vi "Untitled 402.vi"() -> ()   [LabVIEW 2009]
uses:
  <vilib>/addons/_office/excel.llb/Excel Easy Table (str).vi
  <vilib>/Utility/NIReport.llb/NI_report.lvclass
  <vilib>/addons/_office/NI_ReportGenerationToolkit.lvlib
panel:
  out "next cell top-right":cluster{"row":i32, "column":i32}
  out "next cell bottom-left":cluster{"row":i32, "column":i32}
  in  "error in (no error)":errorcluster
  out "Array":i32[][](array[numeric])
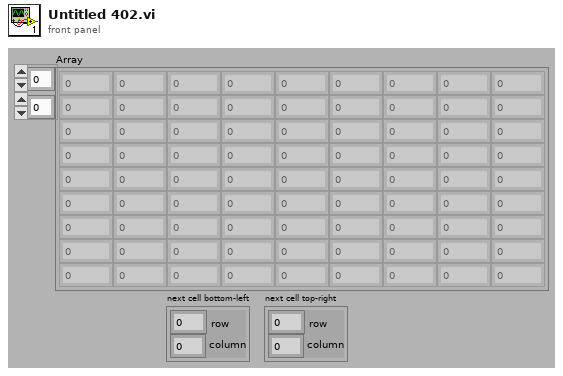
[diagram p1: front panel]
types:
  T1 = enum16{"maximized", "minimized", "normal", "no change"}
  T2 = enum16{"Standard Report", "HTML", "Word", "Excel"}
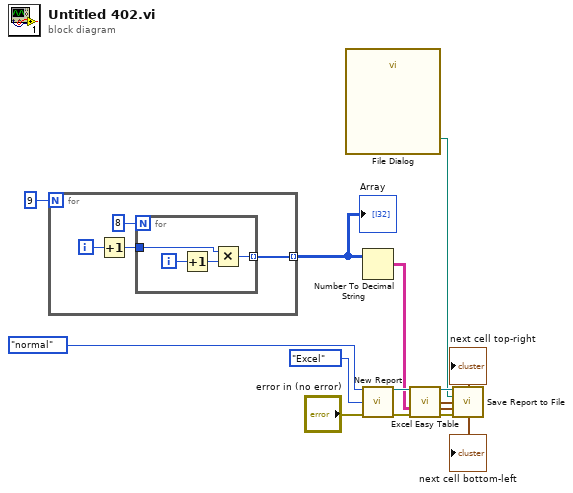
[diagram p0: block diagram]
diagram:
  n1 = for {
    N: 9 -> [_]
    tunnel: [w14] -> w7 mode=indexing
    i -> [w16]
    n2 = Increment(x=w16) -> (x+1=w15:i32)
    n3 = for {
      N: 8 -> [_]
      tunnel: w15 -> [w20]
      tunnel: [w18] -> w14 mode=indexing
      i -> [w21]
      n4 = Increment(x=w21) -> (x+1=w19:i32)
      n5 = Multiply(x=w20, y=w19) -> (x*y=w18:i32)
    }
  }
  "Array" <- w7
  n6 = call "File Dialog"() -> ("selected path"=w8:path)  [unwired: 12 in, 3 out]
  n7 = Number To Decimal String(number=w7) -> (decimal integer string=w6:string[][])  [unwired: 1 in]
  n8 = call <vilib>:"New Report.vi"("window state (normal)"=T1."normal", "report type"=T2."Excel", "error in (no error)"="error in (no error)") -> ("report out"=w12:refnum<class "NI_report.lvclass">, "error out"=w11:errorcluster)  [unwired: 11 in]
  n9 = call-poly <vilib>:"Excel Easy Table.vi"("report in"=w12, "text data"=w6, "error in (no error)"=w11) -> ("report out"=w10:refnum<class "NI_report.lvclass">, "next cell bottom-left"=→"next cell bottom-left":cluster{"row":i32, "column":i32}, "next cell top-right"=→"next cell top-right":cluster{"row":i32, "column":i32}, "error out"=w9:errorcluster)  [unwired: 8 in, 1 out]
  n10 = call-dynamic "Save Report to File.vi"("report in"=w10, "report file path"=w8, "error in (no error)"=w9) -> ()  [unwired: 11 in, 2 out]
